vi "CVT Static Writer.vi"() -> ()   [LabVIEW 2010]
uses:
  _SubVIs/TypeDefs/cvt_Tag Configuration.ctl
  _SubVIs/TypeDefs/cvt_Data Types.ctl
panel:
  in  "stop":bool
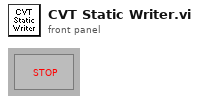
[diagram p1: front panel]
types:
  T1 = typedef "cvt_Tag Configuration.ctl" = cluster{"Name":string, "Data Type":T2, "Array":bool, "Size":u32, "Default":string, "Enum":string[], "Description":string}
  T2 = typedef "cvt_Data Types.ctl" = enum16{"Bool", "U8", "I32", "Double", "String", "Enum"}
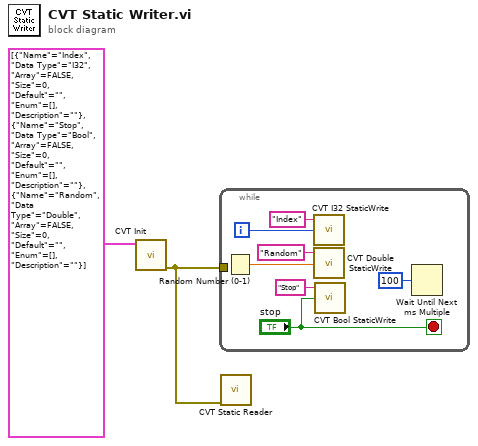
[diagram p0: block diagram]
diagram:
  n1 = call "CVT Init.vi"("Tag List"=T1[] [{"Name"="Index", "Data Type"=enum."I32", "Array"=FALSE, "Size"=0, "Default"="", "Enum"=[], "Description"=""}, {"Name"="Stop", "Data Type"=enum."Bool", "Array"=FALSE, "Size"=0, "Default"="", "Enum"=[], "Description"=""}, {"Name"="Random", "Data Type"=enum."Double", "Array"=FALSE, "Size"=0, "Default"="", "Enum"=[], "Description"=""}]) -> ("error out"=w1:errorcluster)  [unwired: 1 in, 9 out]
  n2 = while {
    tunnel: w1 -> [_]
    i -> [w8]
    stop <- "stop" stop-if-true
    n3 = Random Number (0-1)() -> (number: 0 to 1=w6:dbl)
    n4 = call "CVT I32 StaticWrite.vi"("Value"=w8, "Tag Name"="Index") -> ()  [unwired: 1 in, 3 out]
    n5 = call "CVT Double StaticWrite.vi"("Value"=w6, "Tag Name"="Random") -> ()  [unwired: 1 in, 3 out]
    n6 = call "CVT Bool StaticWrite.vi"("Value"="stop", "Tag Name"="Stop") -> ()  [unwired: 1 in, 3 out]
    n7 = Wait Until Next ms Multiple(millisecond multiple=u32 100) -> ()  [unwired: 1 out]
  }
  n8 = call "CVT Static Reader.vi"("error in (no error)"=w1) -> ()  [unwired: 11 out]
